vi "Front panel.vi"() -> ()   [LabVIEW 2020]
panel:
  in  "Type of Resistor Combination":enum32{"Series", "Parallel"}(radio)
  out "Valid Input":bool
  out "Resistor Value":dbl format="%#_6f"
  in  "Step 10":i16(ring) items=["0 W"=0, "50 W"=50, "100 W"=100, "200 W"=200, "300 W"=300, "500 W"=500, "1000 W"=1000, "2000 W"=2000, "5000 W"=5000, "10000 W"=10000, "12000 W"=12000]
  in  "Step 9":i16(ring) items=["0 W"=0, "50 W"=50, "100 W"=100, "200 W"=200, "300 W"=300, "500 W"=500, "1000 W"=1000, "2000 W"=2000, "5000 W"=5000, "10000 W"=10000, "12000 W"=12000]
  in  "Step 8":i16(ring) items=["0 W"=0, "50 W"=50, "100 W"=100, "200 W"=200, "300 W"=300, "500 W"=500, "1000 W"=1000, "2000 W"=2000, "5000 W"=5000, "10000 W"=10000, "12000 W"=12000]
  in  "Step 7":i16(ring) items=["0 W"=0, "50 W"=50, "100 W"=100, "200 W"=200, "300 W"=300, "500 W"=500, "1000 W"=1000, "2000 W"=2000, "5000 W"=5000, "10000 W"=10000, "12000 W"=12000]
  in  "Step 6":i16(ring) items=["0 W"=0, "50 W"=50, "100 W"=100, "200 W"=200, "300 W"=300, "500 W"=500, "1000 W"=1000, "2000 W"=2000, "5000 W"=5000, "10000 W"=10000, "12000 W"=12000]
  in  "Step 5":i16(ring) items=["0 W"=0, "50 W"=50, "100 W"=100, "200 W"=200, "300 W"=300, "500 W"=500, "1000 W"=1000, "2000 W"=2000, "5000 W"=5000, "10000 W"=10000, "12000 W"=12000]
  in  "Step 4":i16(ring) items=["0 W"=0, "50 W"=50, "100 W"=100, "200 W"=200, "300 W"=300, "500 W"=500, "1000 W"=1000, "2000 W"=2000, "5000 W"=5000, "10000 W"=10000, "12000 W"=12000]
  in  "Step 3":i16(ring) items=["0 W"=0, "50 W"=50, "100 W"=100, "200 W"=200, "300 W"=300, "500 W"=500, "1000 W"=1000, "2000 W"=2000, "5000 W"=5000, "10000 W"=10000, "12000 W"=12000]
  in  "Step 2":i16(ring) items=["0 W"=0, "50 W"=50, "100 W"=100, "200 W"=200, "300 W"=300, "500 W"=500, "1000 W"=1000, "2000 W"=2000, "5000 W"=5000, "10000 W"=10000, "12000 W"=12000]
  in  "Step 1":i16(ring) items=["50 W"=50, "100 W"=100, "200 W"=200, "300 W"=300, "500 W"=500, "1000 W"=1000, "2000 W"=2000, "5000 W"=5000, "10000 W"=10000, "12000 W"=12000]
  in  "DC Voltage":i32(knob) scale=12.0..220.0
  in  "Number of Steps":i16 min=1 max=10 step=1
  in  "Step Type":enum32{"Equal Loading", "Variable Loading"}(radio)
  in  "AC Voltage":enum32{"1 Phase", "3 Phase"}(radio) caption="Only if AC"
  in  "Type of Supply":enum32{"DC Supply", "AC Supply"}(radio)
  in  "Capacity of Load":i16(knob) scale=1.0..12.0
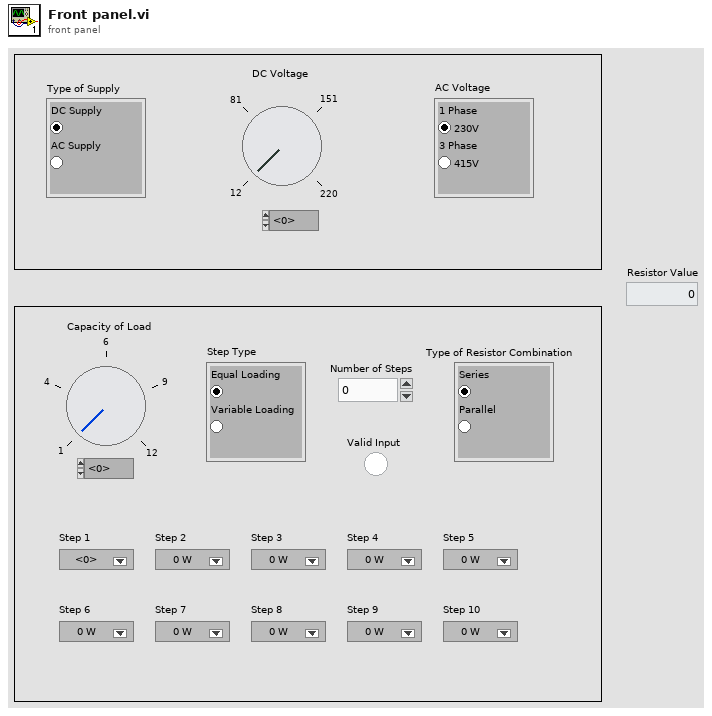
[diagram p1: front panel]
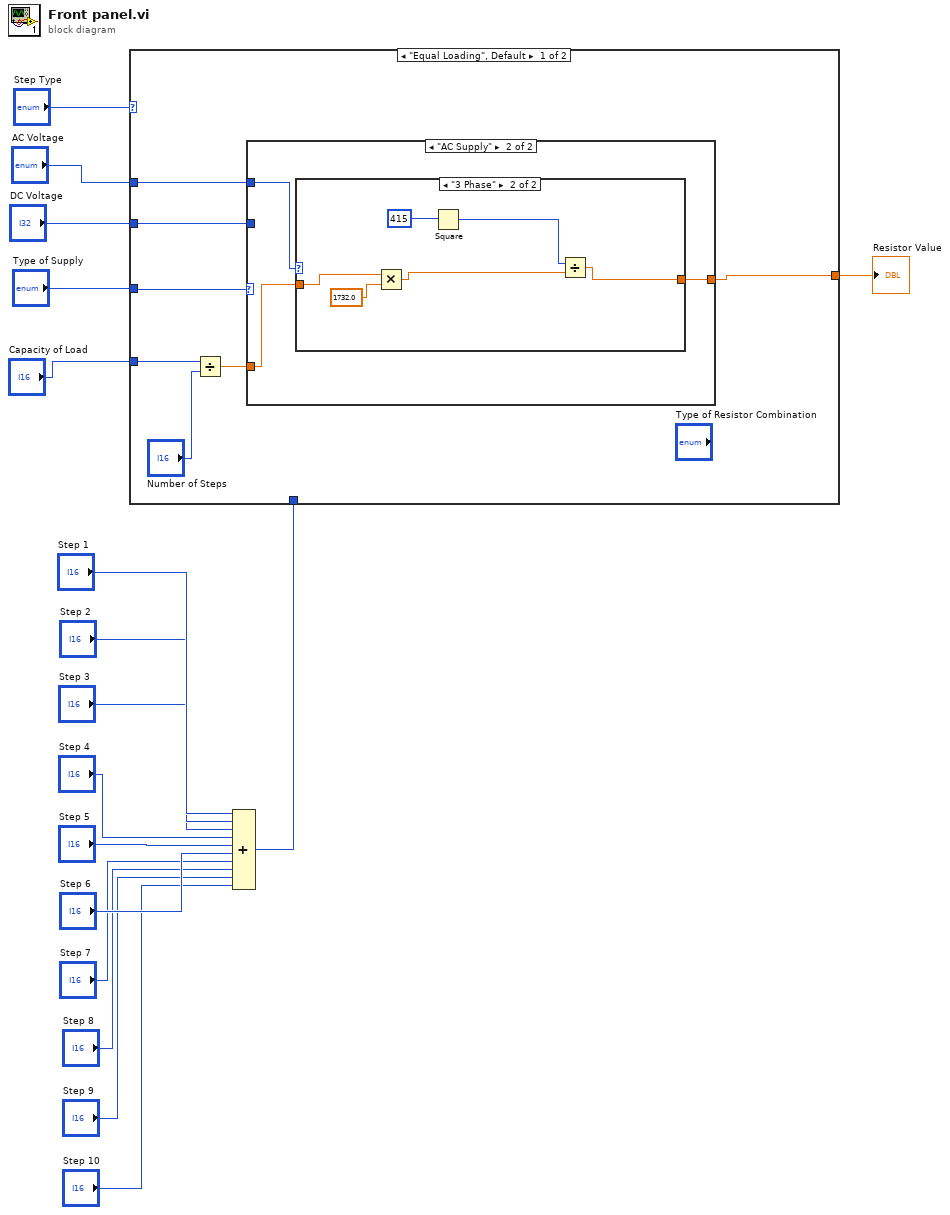
[diagram p0: block diagram]
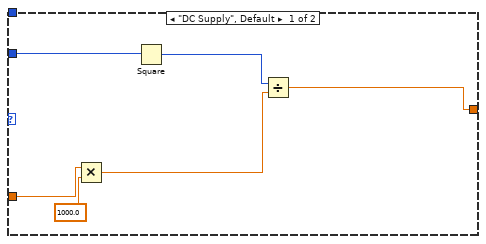
[diagram p2: hidden frame]
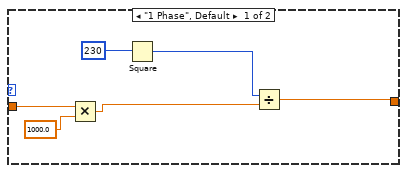
[diagram p3: hidden frame]
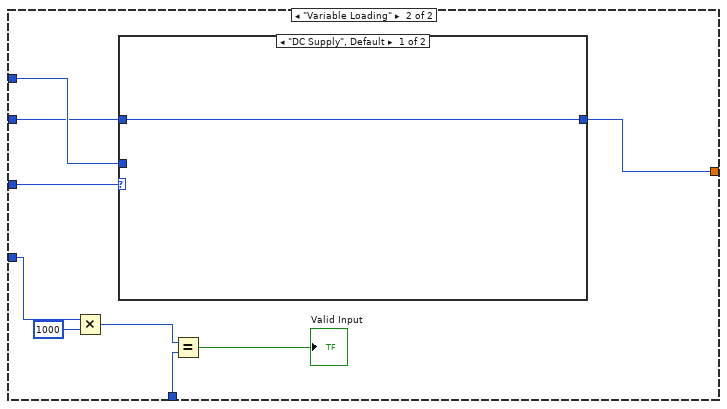
[diagram p4: hidden frame]
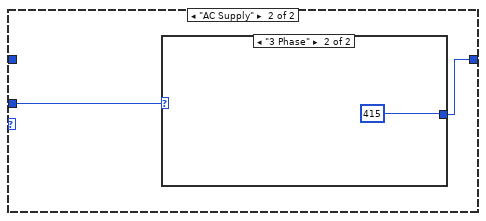
[diagram p5: hidden frame]
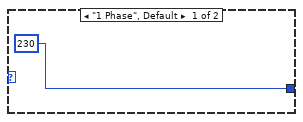
[diagram p6: hidden frame]
diagram:
  n1 = Compound Arithmetic op=ADD("Step 1", "Step 2", "Step 3", "Step 4", "Step 5", "Step 6", "Step 7", "Step 8", "Step 9", "Step 10") -> (w2:i16)
  n2 = case shown="\"Equal Loading\", Default" "Step Type" {
    tunnel: "Type of Supply" -> [w24 w54]
    tunnel: "Capacity of Load" -> [w22 w48]
    tunnel: "AC Voltage" -> [w19 w53]
    tunnel: "DC Voltage" -> [w20 w50]
    tunnel: w2 -> [_ w52]
    tunnel: [w18 w51] -> w1
    frame "Equal Loading", Default {
      n3 = Divide(x=w22, y="Number of Steps") -> (x/y=w21:dbl)
      n4 = case shown="\"AC Supply\"" w24 {
        tunnel: [w25 w33] -> w18
        tunnel: w21 -> [w29 w31]
        tunnel: w20 -> [w28 _]
        tunnel: w19 -> [_ w32]
        frame "DC Supply", Default {
          n5 = Multiply(x=w29, y=1000.0) -> (x*y=w26:dbl)
          n6 = Square(x=w28) -> (x^2=w27:i32)
          n7 = Divide(x=w27, y=w26) -> (x/y=w25:dbl)
        }
        frame "AC Supply" {
          n8 = case shown="\"3 Phase\"" w32 {
            tunnel: [w34 w40] -> w33
            tunnel: w31 -> [w38 w41]
            frame "1 Phase", Default {
              n9 = Multiply(x=w38, y=1000.0) -> (x*y=w35:dbl)
              n10 = Square(x=230) -> (x^2=w36:i32)
              n11 = Divide(x=w36, y=w35) -> (x/y=w34:dbl)
            }
            frame "3 Phase" {
              n12 = Multiply(x=w41, y=1732.0) -> (x*y=w42:dbl)
              n13 = Square(x=415) -> (x^2=w43:i32)
              n14 = Divide(x=w43, y=w42) -> (x/y=w40:dbl)
            }
          }
        }
      }
    }
    frame "Variable Loading" {
      n15 = Multiply(x=w48, y=i16 1000) -> (x*y=w47:i16)
      n16 = case shown="\"DC Supply\", Default" w54 {
        tunnel: w53 -> [_ w57]
        tunnel: [w55 w56] -> w51
        tunnel: w50 -> [w55 _]
        frame "DC Supply", Default {
        }
        frame "AC Supply" {
          n17 = case shown="\"3 Phase\"" w57 {
            tunnel: [230 415] -> w56
            frame "1 Phase", Default {
            }
            frame "3 Phase" {
            }
          }
        }
      }
      n18 = Equal?(x=w47, y=w52) -> (x = y?=→"Valid Input":bool)
    }
  }
  "Resistor Value" <- w1
